vi "h.NET.SetNetworkIpMode.vi"(3 "error in":errorcluster, 4 "Network Mode":T1, 5 "Connection ID":refnum<k5>) -> (0 "error out":errorcluster, 1 "Message":string, 2 "Connection ID":refnum<k5>)   [LabVIEW 2016, in "h.Library.lvlib"]
doc: "Sets the network configuration mode to either static IP addressing or dynamic IP address asignment by DHCP.\n\n<b>Connection ID</b> - is a network connection refnum that uniquely identifies the TCP connection\n<b>Network Mode</b> - sets the network IP addressing mode to either Static (manual) or Dynamic (DHCP)\n<b>error in</b> - describes error conditions that occur before this node runs. This input provides standard error functionality\n<b>Connection ID out</b> - returns the same value as connection ID\n<b>Message</b> - human readable string reporting the outcome of the executed command\n<b>error out</b> - contains error information. This output provides standard error out functionality."
uses:
  h.Library.lvlib
  CTL/h.NET.NetworkMode.ctl
panel:
  # "Hyperion Set Network Configuration Mode"
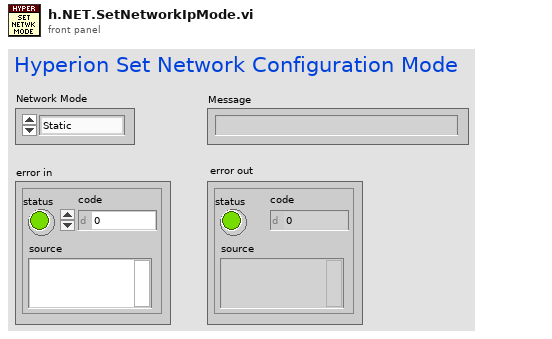
[diagram p1: front panel]
types:
  T1 = typedef "h.Library.lvlib/h.NET.NetworkMode.ctl" = enum8{"Static", "DHCP"}
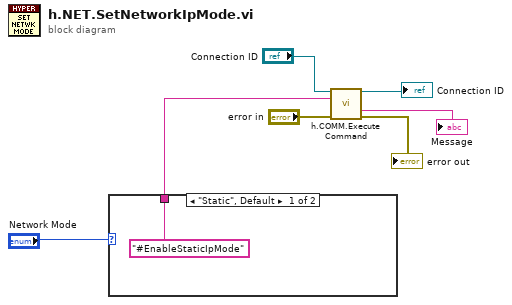
[diagram p0: block diagram]
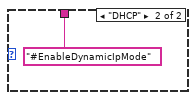
[diagram p2: hidden frame]
diagram:
  n1 = case shown="\"Static\", Default" "Network Mode" {
    tunnel: ["#EnableStaticIpMode" "#EnableDynamicIpMode"] -> w6
    frame "Static", Default {
    }
    frame "DHCP" {
    }
  }
  n2 = call "h.COMM.Execute Command.vi"("Connection ID"="Connection ID", "Command"=w6, "error in"="error in") -> ("Connection ID out"=→"Connection ID":refnum<k5>, "Message"=→"Message":string, "error out"=→"error out":errorcluster)  [unwired: 5 in, 5 out]
